vi "LRU Queue.vi"() -> (3 "LRU Queue":refnum<queue>)   [LabVIEW 2019, in "23.lvlib"]
uses:
  23.lvlib
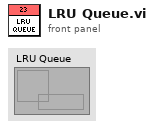
[diagram p1: front panel]
types:
  T1 = cluster{"Stop":bool, "Check":bool, "Key":cluster{"Hallway":string[], "Rooms":string[][]}, "Value":u64, "Check Notifier":refnum<notifier>}
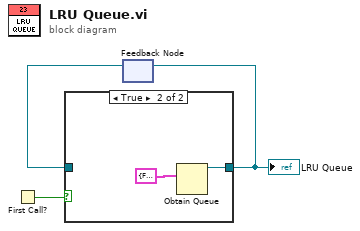
[diagram p0: block diagram]
diagram:
  n1 = First Call?() -> (First Call?: T/F=w1:bool)
  n2 = feedback #1() -> (w2:refnum<queue>)  [unwired: 1 in]
  n3 = case shown="True" w1 {
    tunnel: [w4 w6] -> w3
    tunnel: w2 -> [w4 _]
    frame False {
    }
    frame True {
      n4 = Obtain Queue(element data type=T1 {"Stop"=FALSE, "Check"=FALSE, "Key"={"Hallway"=[], "Rooms"=[]}, "Value"=0, "Check Notifier"=refnum}) -> (queue out=w6:refnum<queue>)  [unwired: 4 in, 2 out]
    }
  }
  "LRU Queue" <- w3
  n5 = feedback-in #1(w3) -> ()
